vi "APSxCreateSensorObject.vi"(8 "error in (no error)":errorcluster caption="错误输入（无错误）", 10 "SensorName":string, 11 "PGIType":enum16{"APSX_PGI_TYPE_1", "APSX_PGI_TYPE_2"}(ring)=enum."APSX_PGI_TYPE_2") -> (0 "error out":errorcluster caption="错误输出", 1 "Message":string, 3 "hSENSOR out":i32)   [LabVIEW 2018]
doc: "该模板用于创建子VI。"
uses:
  APSx.dll/APSx.dll
panel:
  in  "hSENSOR IN":i32
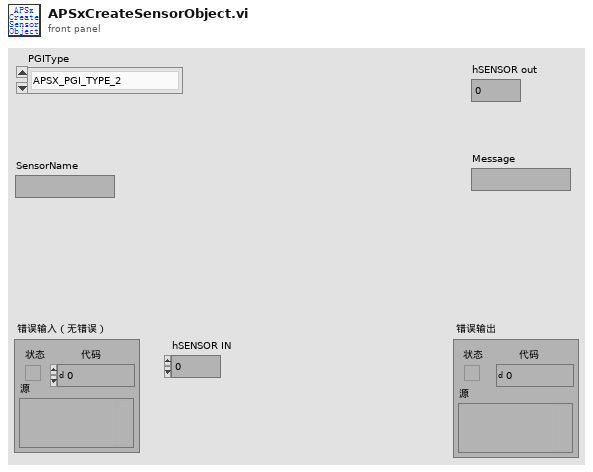
[diagram p1: front panel]
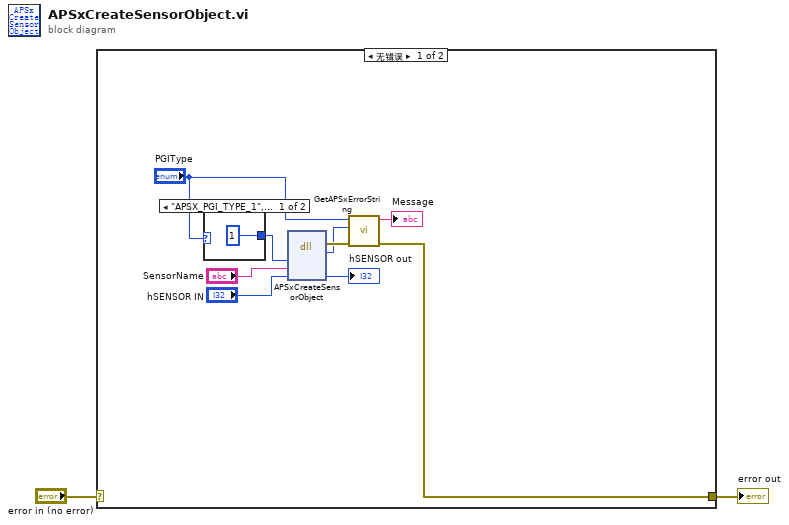
[diagram p0: block diagram]
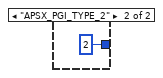
[diagram p2: hidden frame]
diagram:
  n1 = case shown="无错误" "error in (no error)" {
    selector: "error in (no error)" -> [_ w14]
    tunnel: [w6 w14] -> w1
    frame No Error {
      n2 = case shown="\"APSX_PGI_TYPE_1\", 默认" "PGIType" {
        tunnel: [1 2] -> w5
        frame "APSX_PGI_TYPE_1", Default {
        }
        frame "APSX_PGI_TYPE_2" {
        }
      }
      n3 = dll-call lib="PTH2]abs D项目Feng恒隆项目Labview传感器对中台SourcesAPSx.dllAPSx.dll" fn="APSxCreateSensorObject"("PGIType"=w5, "SensorName"="SensorName", "hSENSOR"="hSENSOR IN") -> (error out=w8:errorcluster, "Code"=w7:i32, "hSENSOR"=→"hSENSOR out":i32)  [unwired: 5 in, 1 out]
      n4 = call "GetAPSxErrorString.vi"("error in (no error)"=w8, "ErrorCode"=w7, "PGIType"="PGIType") -> ("error out"=w6:errorcluster, "Message"=→"Message":string)  [unwired: 7 in]
    }
    frame Error {
    }
  }
  "error out" <- w1
